vi "LVH5Rclose (DSet).vi"(6 "error in (no error)":errorcluster, 9 "HDF5 Dataset Region Ref":T1) -> (0 "error out":errorcluster)   [LabVIEW 2017]
doc: "Closes an HDF5 Reference object"
uses:
  <vilib>/UPVI/lvhdf5/reference.llb/H5R Dataset Region Ref.ctl
  <vilib>/UPVI/lvhdf5/h5helper.dll
panel:
  # "LVHDF5 Toolkit\nCopyright (c) 2005-2013 by Jason D. Sommerville\nCopyright (c) 2014 by UPVI, LLC.\n\nThis use and distribution of this file is governed by the terms found in \nLICENSE.txt distributed with this toolkit and installed at\n <user.lib>\\_lvhdf5\\LICENSE.txt"
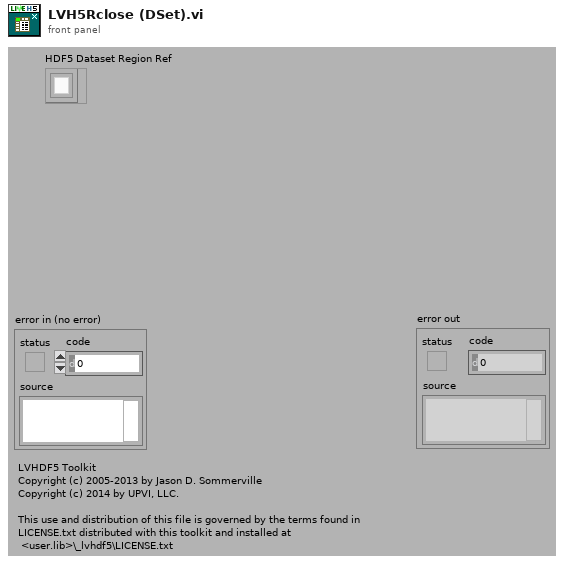
[diagram p1: front panel]
types:
  T1 = typedef "H5R Dataset Region Ref.ctl" = refnum<k1>
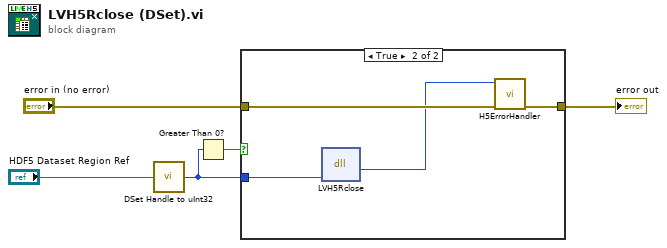
[diagram p0: block diagram]
diagram:
  n1 = call <vilib>:"DSet Handle to uInt32.vi"("HDF5 Reference Type"="HDF5 Dataset Region Ref") -> ("Handle"=w1:u32)
  n2 = Greater Than 0?(x=w1) -> (x > 0?=w3:bool)
  n3 = case shown="True" w3 {
    tunnel: "error in (no error)" -> [w6 w10]
    tunnel: [w6 w9] -> w4
    tunnel: w1 -> [_ w7]
    frame False {
    }
    frame True {
      n4 = dll-call lib="C:/Program Files/National Instruments/LabVIEW 2017/vi.lib/UPVI/lvhdf5/h5helper.dll" fn="LVH5Rclose"("attr_id"=w7) -> (w8:i32)  [unwired: 4 in, 2 out]
      n5 = call <vilib>:"H5ErrorHandler.vi"("error in (no error)"=w10, "herr_t"=w8) -> ("error out"=w9:errorcluster)  [unwired: 3 in, 4 out]
    }
  }
  "error out" <- w4
